vi "SE Mask Offset Outer List Stop Configure Abs Amp Limit Couple Enabled.vi"(8 "error in (no error)":errorcluster {"code" format="%.0x"}, 9 "State":u16[](array[numeric]), 11 "instrument handle":refnum<k15>) -> (0 "error out":errorcluster {"code" format="%.0x"}, 3 "instrument handle out":refnum<k15>)   [LabVIEW 2021, in "Keysight XSAnVMA.lvlib"]
doc: "Enable or disable the absolute power level limit at the stop frequency for the selected offset."
uses:
  <instrlib>/Keysight XSAnVMA/Keysight XSAnVMA.lvlib
  KtXSAnVMA_64.dll
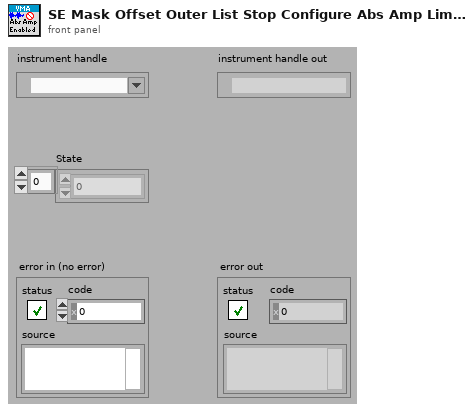
[diagram p1: front panel]
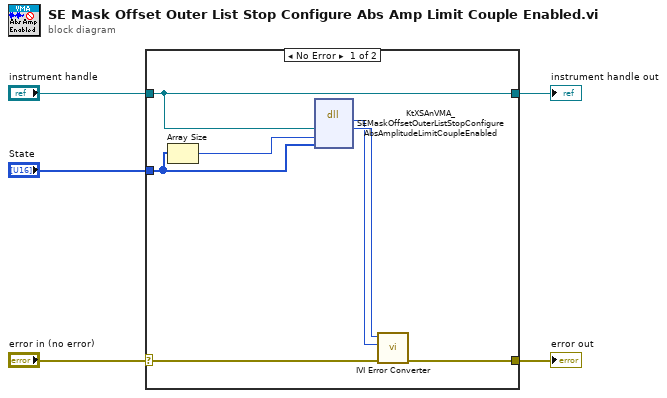
[diagram p0: block diagram]
diagram:
  n1 = case shown="No Error" "error in (no error)" {
    selector: "error in (no error)" -> [w10 w14]
    tunnel: [w9 w14] -> w5
    tunnel: "instrument handle" -> [w8 w13]
    tunnel: "State" -> [w6 _]
    tunnel: [w8 w13] -> w1
    frame No Error {
      n2 = Array Size(array=w6) -> (size(s)=w7:i32)
      n3 = dll-call lib="KtXSAnVMA**.dll" fn="KtXSAnVMA_SEMaskOffsetOuterListStopConfigureAbsAmplitudeLimitCoupleEnabled"("Vi"=w8, "StateBufferSize"=w7, "State"=w6) -> (w11:i32, "Vi"=w12:u32)  [unwired: 5 in, 2 out]
      n4 = call <instrlib>:"IVI Error Converter.vi"("error in (no error)"=w10, "IVI error code (0)"=w11, "instrument handle"=w12) -> ("error out"=w9:errorcluster)  [unwired: 7 in, 1 out]
    }
    frame Error {
    }
  }
  "error out" <- w5
  "instrument handle out" <- w1
